vi "GetPSUStatus.vi"(8 "error in (no error)":errorcluster, 11 "PSU_N87 in":refnum<class "PSU_N67.lvclass">) -> (0 "error out":errorcluster, 1 "OCP Tripped":bool, 2 "OVP Tripped":bool, 3 "PSU_N87 out":refnum<class "PSU_N67.lvclass">, 4 "Current (A)":dbl, 5 "Voltage (V)":dbl)   [LabVIEW 2014, in "PSU_N67.lvclass"]
uses:
  PSU_N67.lvclass
  PSU.lvclass/PSU.ctl
  PSU_N67.lvclass/PSU_N67.ctl
  Read Channel.vi
  <instrlib>/Agilent N6700 Series/Agilent N6700 Series.lvlib
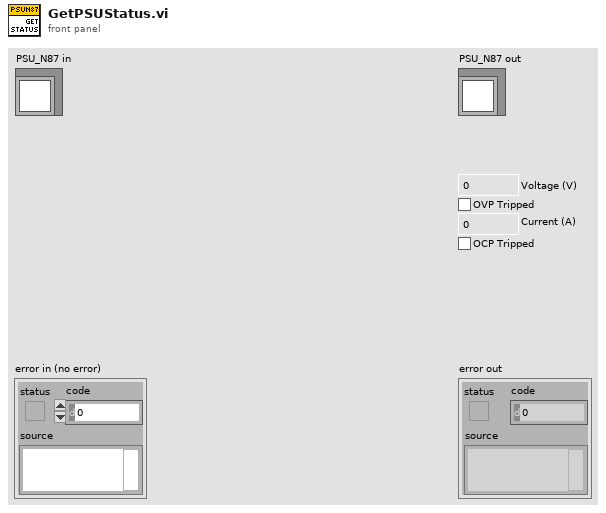
[diagram p1: front panel]
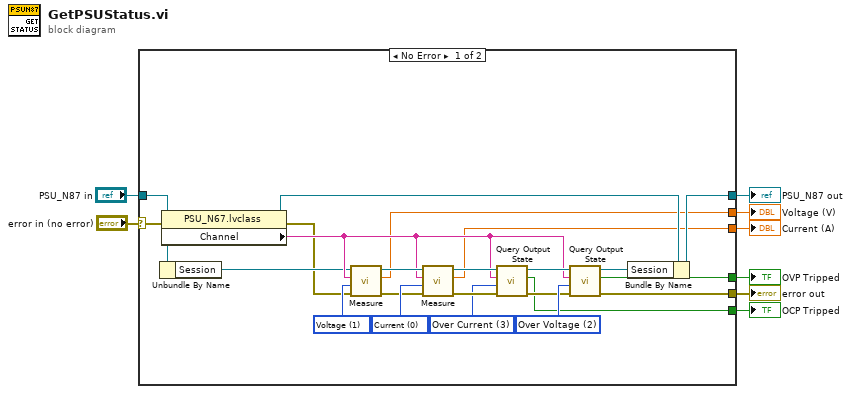
[diagram p0: block diagram]
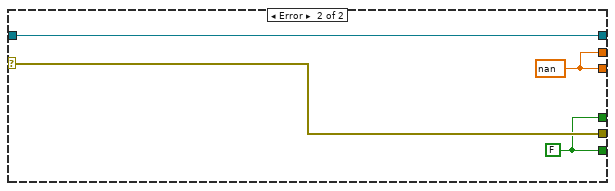
[diagram p2: hidden frame]
diagram:
  n1 = case shown="No Error" "error in (no error)" {
    selector: "error in (no error)" -> [w17 w35]
    tunnel: "PSU_N87 in" -> [w21 w34]
    tunnel: [w11 w33] -> w7
    tunnel: [w12 w33] -> w6
    tunnel: [w13 w32] -> w1
    tunnel: [w9 w32] -> w2
    tunnel: [w10 w35] -> w5
    tunnel: [w15 w34] -> w3
    frame No Error {
      w30 = 0 items=["Current", "Voltage", "Power"] ("Measurement Type (1: Voltage)")
      w26 = 2 items=["Constant Voltage"=0, "Constant Current"=1, "Unregulated"=4, "Over Voltage"=2, "Over Current"=3] ("Output State (0: Constant Voltage)")
      w23 = 3 items=["Constant Voltage"=0, "Constant Current"=1, "Unregulated"=4, "Over Voltage"=2, "Over Current"=3] ("Output State (0: Constant Voltage)")
      w22 = 1 items=["Current", "Voltage", "Power"] ("Measurement Type (1: Voltage)")
      n2 = Unbundle By Name(w21) -> ("Session"=w19:refnum<visa-resource-name>)
      n3 = property class="PSU_N67.lvclass"(reference=w21, error in=w17) -> (reference out=w14:refnum<class "PSU_N67.lvclass">, error out=w16:errorcluster, "Channel"=w20:string)
      n4 = call <instrlib>:"Measure.vi"("error in (no error)"=w16, "Measurement Type (1: Voltage)"=w22, "Channel Name (1)"=w20, "VISA resource name"=w19) -> ("error out"=w27:errorcluster, "Measurement"=w11:dbl, "VISA resource name out"=w29:refnum<visa-resource-name>)  [unwired: 5 in]
      n5 = call <instrlib>:"Measure.vi"("error in (no error)"=w27, "Measurement Type (1: Voltage)"=w30, "Channel Name (1)"=w20, "VISA resource name"=w29) -> ("error out"=w28:errorcluster, "Measurement"=w12:dbl, "VISA resource name out"=w31:refnum<visa-resource-name>)  [unwired: 5 in]
      n6 = call <instrlib>:"Query Output State.vi"("error in (no error)"=w28, "Output State (0: Constant Voltage)"=w23, "Channel Name (1)"=w20, "VISA resource name"=w31) -> ("error out"=w24:errorcluster, "In State"=w9:bool, "VISA resource name out"=w25:refnum<visa-resource-name>)  [unwired: 5 in]
      n7 = call <instrlib>:"Query Output State.vi"("error in (no error)"=w24, "Output State (0: Constant Voltage)"=w26, "Channel Name (1)"=w20, "VISA resource name"=w25) -> ("error out"=w10:errorcluster, "In State"=w13:bool, "VISA resource name out"=w18:refnum<visa-resource-name>)  [unwired: 5 in]
      n8 = Bundle By Name(cluster=w14, "Session"=w18) -> (w15:refnum<class "PSU_N67.lvclass">)
    }
    frame Error {
      w32 = FALSE ("OVP Tripped?")
      w33 = nan ("Actual Voltage Level (V)")
    }
  }
  "error out" <- w5
  "PSU_N87 out" <- w3
  "Voltage (V)" <- w7
  "Current (A)" <- w6
  "OCP Tripped" <- w2
  "OVP Tripped" <- w1
